vi "verify temperature.vi"(8 "error in (no error)":errorcluster, 11 "Simulated Camera in":refnum<class "Sim_CCD.lvclass">) -> (0 "error out":errorcluster, 3 "Simulated Camera out":refnum<class "Sim_CCD.lvclass">)   [LabVIEW 2018, in "Sim_CCD.lvclass"]
uses:
  Sim_CCD.lvclass
  Sim_CCD.lvclass/Sim_CCD.ctl
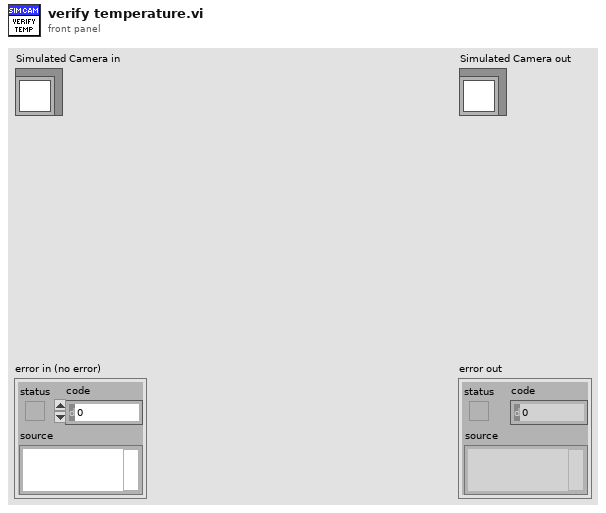
[diagram p1: front panel]
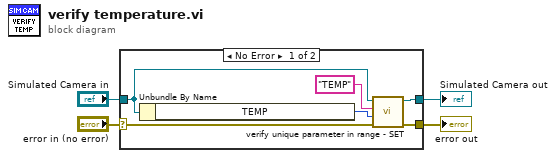
[diagram p0: block diagram]
diagram:
  n1 = case shown="No Error" "error in (no error)" {
    selector: "error in (no error)" -> [w8 w12]
    tunnel: [w9 w12] -> w3
    tunnel: [w10 w11] -> w1
    tunnel: "Simulated Camera in" -> [w6 w11]
    frame No Error {
      n2 = Unbundle By Name(w6) -> ("TEMP"=w5:i32)
      n3 = call "verify unique parameter in range - SET.vi"("error in (no error)"=w8, "value"=w5, "parameter name"="TEMP", "Simulated_CCD_Camera in"=w6) -> ("error out"=w9:errorcluster, "Simulated_CCD_Camera out"=w10:refnum<class "Sim_CCD.lvclass">)  [unwired: 6 in]
    }
    frame Error {
    }
  }
  "error out" <- w3
  "Simulated Camera out" <- w1
